vi "c_Update shutter.vi"() -> (1 "Case Label":T1)   [LabVIEW 2023, in "UI Cam Basler.lvclass"]
uses:
  <vilib>/addons/_Workers/Library/Case Label.ctl
  UI Cam Basler.lvclass
  UI Cam Basler.lvclass/UI Cam Basler.ctl
  <vilib>/addons/_Workers/Library/Workers.lvlib
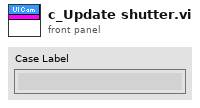
[diagram p1: front panel]
types:
  T1 = typedef "Workers.lvlib/Case Label.ctl" = string
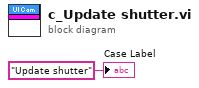
[diagram p0: block diagram]
diagram:
  "Case Label" <- T1 "Update shutter" ("Case Label")
